vi "Vision Research Phantom Series PhFile PhDestroyCine.vi"(1 "CH in":u32, 5 "Error In (no error)":errorcluster) -> (15 "CH out":u32, 19 "Error Out":errorcluster)   [LabVIEW 2013, in "VRI.lvlib"]
doc: "PhFile.dll\n\nPhDestroyCine\nHRESULT PhDestroyCine(CINEHANDLE CH);\n\nParameters Description\nCH(in) Handle of the file cine.\nReturn HRESULT (0 = Ok)\nComments This function should be called in order to \n free the resources allocated in phfile.dll\n for the cine structure.\n\n\nWritten by:\nBLOOMY CONTROLS, INC\nWINDSOR, CT 06095, USA\n860-298-9925\nwww.bloomy.com\nV1.0.0\nMay, 2004"
uses:
  VRI.lvlib
  Phantom DLLs/PhFile.Dll
panel:
  # "For instructions on the use of this VI, press Ctrl+H to display the help window and move the mouse over the icon, controls, and indicators"
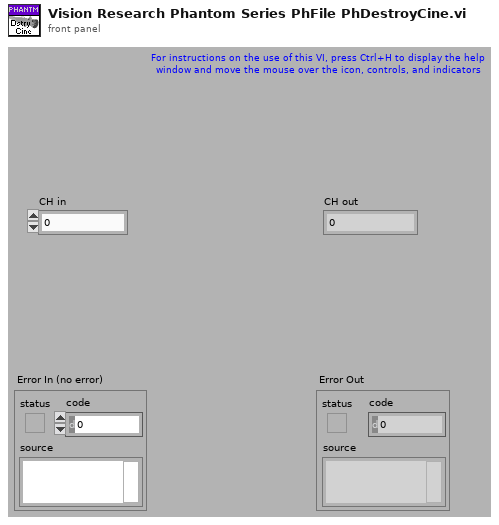
[diagram p1: front panel]
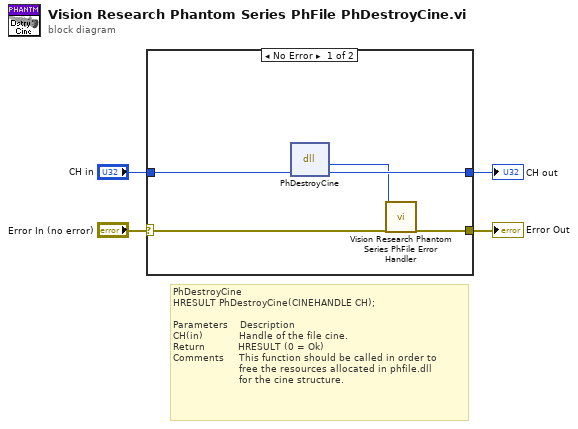
[diagram p0: block diagram]
diagram:
  # "PhDestroyCine\nHRESULT PhDestroyCine(CINEHANDLE CH);\n\nParameters    Description\nCH(in)            Handle of the file cine.\nReturn           HRESULT (0 = Ok)\nComments     This function should be called in order to \n                      free the resources allocated in phfile.dll\n                      for the cine structure."
  n1 = case shown="No Error" "Error In (no error)" {
    selector: "Error In (no error)" -> [w9 w11]
    tunnel: [w8 w11] -> w3
    tunnel: "CH in" -> [w7 w10]
    tunnel: [w6 w10] -> w1
    frame No Error {
      n2 = dll-call lib="C:/Projects/SDK/64-bit/Vision Research Phantom Series Labview Driver/Phantom DLLs/PhFile.dll" fn="PhDestroyCine"("CH"=w7) -> ("HRESULT"=w5:i32, "CH"=w6:u32)  [unwired: 3 in, 2 out]
      n3 = call "Vision Research Phantom Series PhFile Error Handler.vi"("Error Code (0)"=w5, "Error In (no error)"=w9) -> ("Error Out"=w8:errorcluster)  [unwired: 17 out]
    }
    frame Error {
    }
  }
  "Error Out" <- w3
  "CH out" <- w1
